vi "el2clust.vi"(4 "error out":errorcluster, 5 "Cluster in":T1, 6 "type":string, 7 "element":string) -> (0 "error out 2":errorcluster, 2 "Cluster":T1)   [LabVIEW 2010]
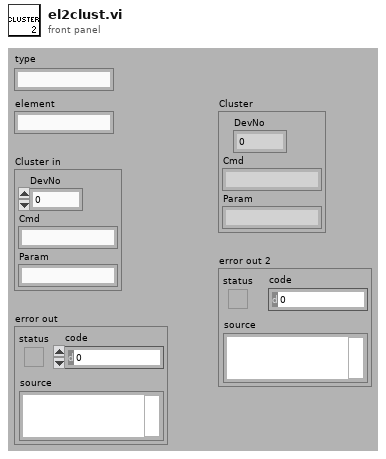
[diagram p1: front panel]
types:
  T1 = cluster{"DevNo":i32, "Cmd":string, "Param":string}
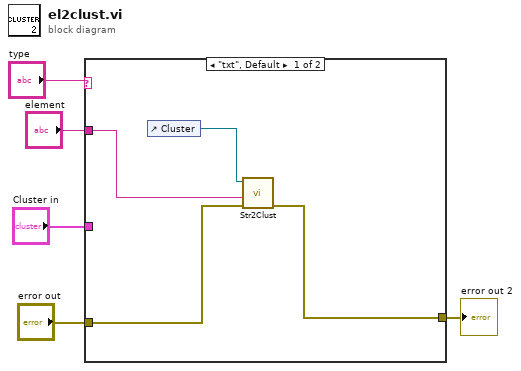
[diagram p0: block diagram]
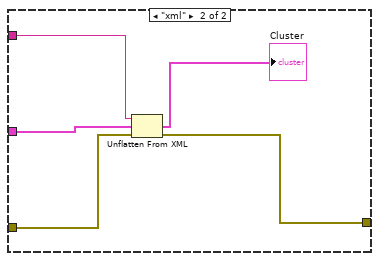
[diagram p2: hidden frame]
diagram:
  n1 = case shown="\"txt\", Default" "type" {
    tunnel: "error out" -> [w9 w14]
    tunnel: "element" -> [w6 w13]
    tunnel: [w8 w12] -> w3
    tunnel: "Cluster in" -> [_ w11]
    frame "txt", Default {
      n2 = control-ref of="Cluster"() -> (w7:refnum<vi>)
      n3 = call "Str2Clust.vi"("error in (no error)"=w9, "String"=w6, "Clust Refnum"=w7) -> ("error out"=w8:errorcluster)  [unwired: 4 in]
    }
    frame "xml" {
      n4 = Unflatten From XML(xml string=w13, type=w11, error in (no error)=w14) -> (value=→"Cluster":T1, error out=w12:errorcluster)
    }
  }
  "error out 2" <- w3
